vi "ModbusResponse.vi"(0 "Modbus Frame":string) -> (1 "Function Code":u8 format="%1x", 2 "Byte Count":i16, 3 "Data":dbl)   [LabVIEW 2016]
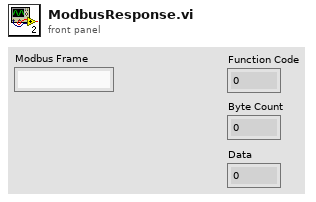
[diagram p1: front panel]
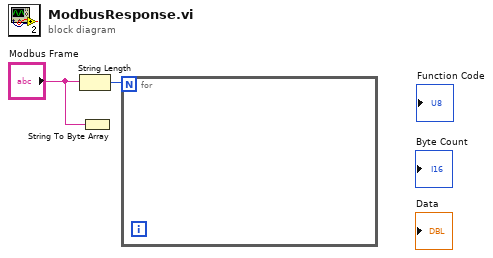
[diagram p0: block diagram]
diagram:
  n1 = String Length(string="Modbus Frame") -> (length=w2:i32)
  n2 = String To Byte Array(string="Modbus Frame") -> ()  [unwired: 1 out]
  n3 = for {
    N: w2 -> [_]
  }
